vi "Request Clear Multiple DTCs.vi"(6 "Command":string, 7 "Ignore Response":bool, 8 "error in":errorcluster, 9 "Address":string, 10 "Lookup Table":variant, 11 "connection info":T3) -> (0 "error out":errorcluster, 2 "Lookup Table":variant, 3 "connection info":T3, 4 "Error Array":T1[](array[typedef]))   [LabVIEW 2019, in "J1939 Addon Shared.lvlib"]
uses:
  J1939 Addon Shared.lvlib
  <vilib>/NI/STM/TCP/TCP Connection Info.ctl
  <vilib>/NI/STM/SubVIs/MetaDataElement.ctl
  Types/Error Cluster.ctl
  Types/Error Types.ctl
  Types/Address Lookup Table Data.ctl
  Types/Request Message.ctl
  <vilib>/NI/STM/NI STM.lvlib
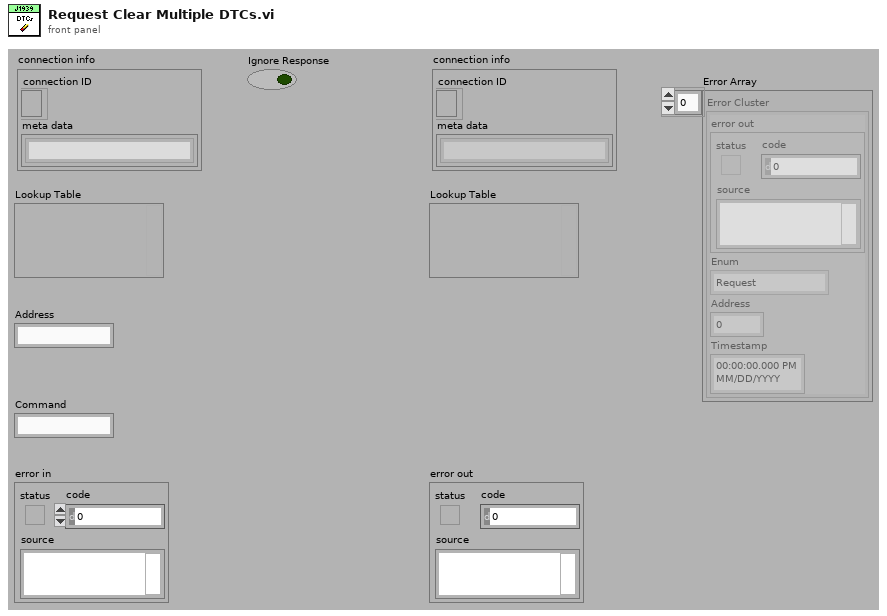
[diagram p1: front panel]
types:
  T1 = typedef "J1939 Addon Shared.lvlib/Error Cluster.ctl" = cluster{"error out":errorcluster, "Enum":T2, "Address":u8, "Timestamp":timestamp}
  T2 = typedef "J1939 Addon Shared.lvlib/Error Types.ctl" = enum16{"Request", "RAW Generation", "Clear Active DTCs", "Clear Previous DTCs", "Addresses", "TLAs", "Get Active DTCs", "Get Previous DTCs", "TCP Connection"}
  T3 = typedef "NI STM.lvlib/TCP Connection Info.ctl" = cluster{"connection ID":refnum<k5>, "meta data":T4[]}
  T4 = typedef "NI STM.lvlib/MetaDataElement.ctl" = string
  T5 = typedef "J1939 Addon Shared.lvlib/Address Lookup Table Data.ctl" = cluster{"Name":u8[], "Address":u8}
  T6 = typedef "J1939 Addon Shared.lvlib/Request Message.ctl" = cluster{"PGN":u32, "DA":u8, "Ignore Response":bool}
  T7 = typedef "XNET Frame CAN.ctl" = cluster{"timestamp":timestamp, "payload":u8[], "identifier":u32, "type":T8, "extended?":bool, "echo?":bool}
  T8 = typedef "XNET Frame Type CAN.ctl" = u8
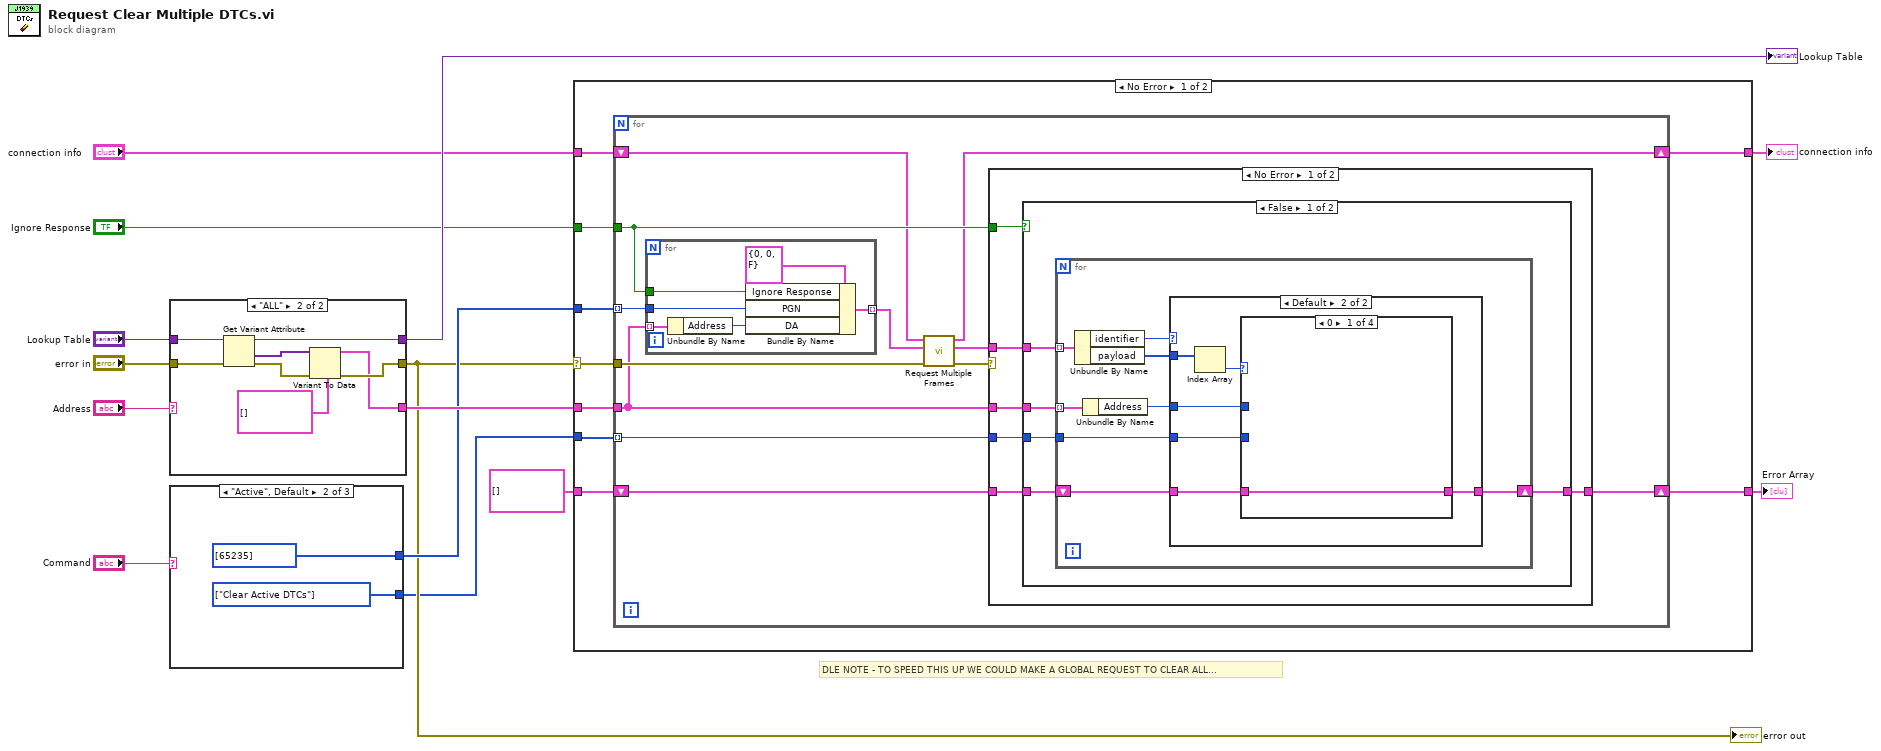
[diagram p0: block diagram]
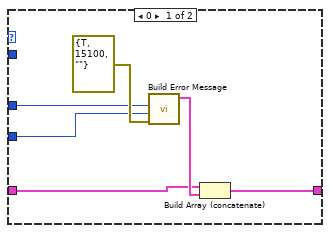
[diagram p2: hidden frame]
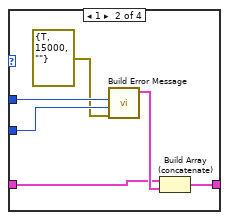
[diagram p3: hidden frame]
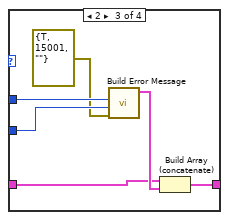
[diagram p4: hidden frame]
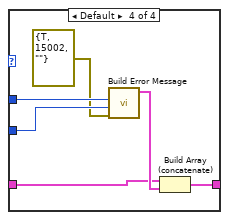
[diagram p5: hidden frame]
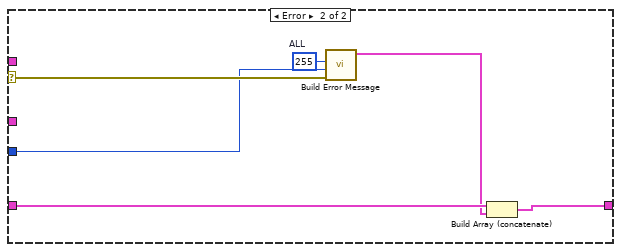
[diagram p7: hidden frame]
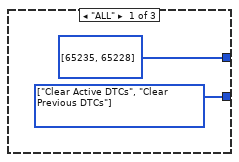
[diagram p9: hidden frame]
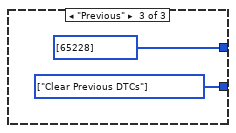
[diagram p10: hidden frame]
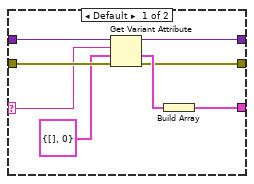
[diagram p11: hidden frame]
diagram:
  # "DLE NOTE - TO SPEED THIS UP WE COULD MAKE A GLOBAL REQUEST TO CLEAR ALL..."
  n1 = case shown="\"ALL\"" "Address" {
    selector: "Address" -> [w17 _]
    tunnel: [w16 w23] -> w14
    tunnel: [w21 w30] -> w13
    tunnel: "Lookup Table" -> [w20 w29]
    tunnel: "error in" -> [w19 w28]
    tunnel: [w18 w26] -> w4
    frame Default {
      n2 = Get Variant Attribute(Variant=w20, name=w17, default value (empty Variant)=T5 {"Name"=[], "Address"=0} ("Data"), error in=w19) -> (duplicate Variant=w21:variant, value=w22:T5, error out=w18:errorcluster)  [unwired: 1 out]
      n3 = Build Array(w22) -> (w16:T5[])
    }
    frame "ALL" {
      n4 = Get Variant Attribute(Variant=w29, error in=w28) -> (duplicate Variant=w30:variant, values=w24:variant[], error out=w27:errorcluster)  [unwired: 2 in, 1 out]
      n5 = Variant To Data(error in=w27, type=T5[] [], Variant=w24) -> (data=w23:T5[], error out=w26:errorcluster)
    }
  }
  "Lookup Table" <- w13
  "error out" <- w4
  n6 = case shown="\"Active\", Default" "Command" {
    tunnel: [u32[] [65235, 65228] u32[] [65235] u32[] [65228]] -> w7
    tunnel: [w31 w33 w35] -> w2
    frame "ALL" {
      w31 = T2[] [enum."Clear Active DTCs", enum."Clear Previous DTCs"] items=["Request", "RAW Generation", "Clear Active DTCs", "Clear Previous DTCs", "Addresses", "TLAs", "Get Active DTCs", "Get Previous DTCs", "TCP Connection"]
    }
    frame "Active", Default {
      w33 = T2[] [enum."Clear Active DTCs"] items=["Request", "RAW Generation", "Clear Active DTCs", "Clear Previous DTCs", "Addresses", "TLAs", "Get Active DTCs", "Get Previous DTCs", "TCP Connection"]
    }
    frame "Previous" {
      w35 = T2[] [enum."Clear Previous DTCs"] items=["Request", "RAW Generation", "Clear Active DTCs", "Clear Previous DTCs", "Addresses", "TLAs", "Get Active DTCs", "Get Previous DTCs", "TCP Connection"]
    }
  }
  n7 = case shown="No Error" w4 {
    selector: w4 -> [w39 _]
    tunnel: w14 -> [w45 _]
    tunnel: [w44 w122] -> w11
    tunnel: "connection info" -> [w43 w122]
    tunnel: w7 -> [w42 _]
    tunnel: T1[] [] -> [w41 w121]
    tunnel: [w40 w121] -> w3
    tunnel: w2 -> [w38 _]
    tunnel: "Ignore Response" -> [w37 _]
    frame No Error {
      n8 = for {
        tunnel: w39 -> [w52]
        tunnel: w45 -> [w46]
        shift-right: [w47] -> w44
        shift-left: w43 -> [w50]
        tunnel: w42 -> [w54] mode=indexing
        shift-right: [w56] -> w40
        shift-left: w41 -> [w57]
        tunnel: w38 -> [w55] mode=indexing
        tunnel: w37 -> [w53]
        n9 = for {
          tunnel: w46 -> [w62] mode=indexing
          tunnel: [w60] -> w49 mode=indexing
          tunnel: w54 -> [w59]
          tunnel: w53 -> [w58]
          n10 = Unbundle By Name(w62) -> ("Address"=w61:u8)
          n11 = Bundle By Name(cluster=T6 {"PGN"=0, "DA"=0, "Ignore Response"=FALSE} ("Cluster"), "Ignore Response"=w58, "PGN"=w59, "DA"=w61) -> (w60:T6)
        }
        n12 = call "Request Multiple Frames.vi"("error in (no error)"=w52, "Requests"=w49, "connection info"=w50) -> ("error out"=w51:errorcluster, "Response Frames"=w48:T7[], "connection info"=w47:T3)  [unwired: 6 in]
        n13 = case shown="No Error" w51 {
          selector: w51 -> [_ w118]
          tunnel: w48 -> [w69 _]
          tunnel: w57 -> [w68 w120]
          tunnel: [w66 w119] -> w56
          tunnel: w55 -> [w67 w117]
          tunnel: w53 -> [w65 _]
          tunnel: w46 -> [w64 _]
          frame No Error {
            n14 = case shown="False" w65 {
              tunnel: w69 -> [w74 _]
              tunnel: w68 -> [w73 w114]
              tunnel: w67 -> [w72 _]
              tunnel: [w71 w114] -> w66
              tunnel: w64 -> [w70 _]
              frame False {
                n15 = for {
                  tunnel: w74 -> [w82] mode=indexing
                  tunnel: w72 -> [w78]
                  tunnel: w70 -> [w76] mode=indexing
                  shift-right: [w77] -> w71
                  shift-left: w73 -> [w79]
                  n16 = Unbundle By Name(w82) -> ("identifier"=w81:u32, "payload"=w80:u8[])
                  n17 = Unbundle By Name(w76) -> ("Address"=w75:u8)
                  n18 = case shown="Default" w81 {
                    tunnel: w80 -> [_ w94]
                    tunnel: w79 -> [w86 w90]
                    tunnel: w75 -> [w83 w92]
                    tunnel: w78 -> [w84 w91]
                    tunnel: [w85 w89] -> w77
                    frame 0 {
                      n19 = call "Build Error Message.vi"("error IO"=errorcluster {"status"=TRUE, "code"=15100, "source"=""}, "Enum"=w84, "Address"=w83) -> ("Error Cluster"=w87:T1)  [unwired: 8 in]
                      n20 = Build Array (concatenate)(w86, w87) -> (w85:T1[])
                    }
                    frame Default {
                      n21 = Index Array(array=w94) -> (element=w93:u8)  [unwired: 1 in]
                      n22 = case shown="0" w93 {
                        tunnel: w92 -> [_ w101 w107 w113]
                        tunnel: w91 -> [_ w100 w106 w112]
                        tunnel: w90 -> [w95 w97 w103 w109]
                        tunnel: [w95 w96 w102 w108] -> w89
                        frame 0 {
                        }
                        frame 1 {
                          n23 = call "Build Error Message.vi"("error IO"=errorcluster {"status"=TRUE, "code"=15000, "source"=""}, "Enum"=w100, "Address"=w101) -> ("Error Cluster"=w98:T1)  [unwired: 8 in]
                          n24 = Build Array (concatenate)(w97, w98) -> (w96:T1[])
                        }
                        frame 2 {
                          n25 = call "Build Error Message.vi"("error IO"=errorcluster {"status"=TRUE, "code"=15001, "source"=""}, "Enum"=w106, "Address"=w107) -> ("Error Cluster"=w104:T1)  [unwired: 8 in]
                          n26 = Build Array (concatenate)(w103, w104) -> (w102:T1[])
                        }
                        frame Default {
                          n27 = call "Build Error Message.vi"("error IO"=errorcluster {"status"=TRUE, "code"=15002, "source"=""}, "Enum"=w112, "Address"=w113) -> ("Error Cluster"=w110:T1)  [unwired: 8 in]
                          n28 = Build Array (concatenate)(w109, w110) -> (w108:T1[])
                        }
                      }
                    }
                  }
                }
              }
              frame True {
              }
            }
          }
          frame Error {
            w115 = u8 255  # ALL
            n29 = call "Build Error Message.vi"("error IO"=w118, "Enum"=w117, "Address"=w115) -> ("Error Cluster"=w116:T1)  [unwired: 8 in]
            n30 = Build Array (concatenate)(w120, w116) -> (w119:T1[])
          }
        }
      }
    }
    frame Error {
    }
  }
  "connection info" <- w11
  "Error Array" <- w3
